vi "ZernikeModeAmp_RangeLimiter_v02.vi"(1 "x_in":dbl[](array[numeric]), 2 "Base Values":dbl[](array[numeric])) -> (0 "x_out":dbl[](array[numeric]))   [LabVIEW 2015]
panel:
  out "x_in relative":dbl[](array[numeric])
  in  "Limit":dbl[](array[numeric])=[1.0, 1.0, 1.0, 1.0, 1.5, 1.0, 1.5, 1.5, 1.0, 1.0, 1.0, 1.0, 1.0, 1.0, 1.0, 1.0, 1.0, 1.0, 1.0, 1.0, 1.0, 0.6, 1.0, 1.0, 1.0, 1.0, 1.0, 1.0, 1.0]
  # "piston"
  # "tip"
  # "tilt"
  # "defocus"
  # "astigmatism (oblique)"
  # "astigmatism (vertical)"
  # "coma"
  # "coma"
  # "trefoil (vertical)"
  # "trefoil (horizontal)"
  # "1st order Spherical Aberration"
  # "2nd order Astigmatism"
  # "2nd order Astigmatism"
  # "quadrafoil"
  # "quadrafoil"
  # "2nd order coma"
  # "2nd order coma"
  # "2nd order Spherical Aberration"
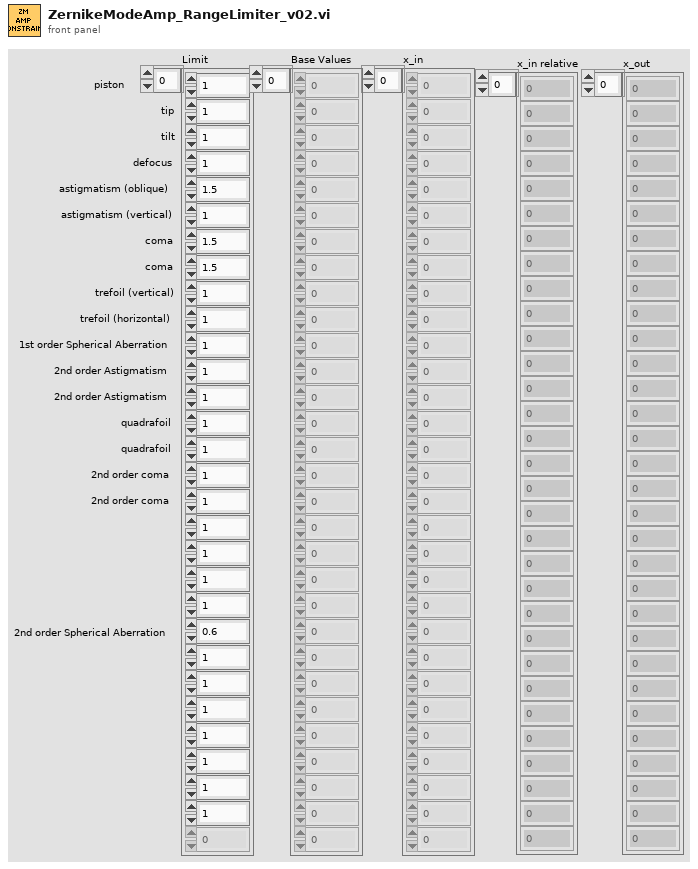
[diagram p1: front panel]
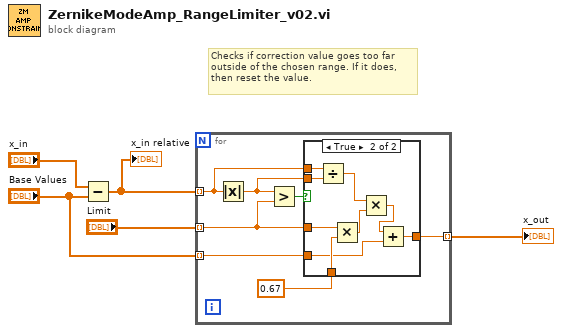
[diagram p0: block diagram]
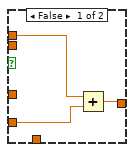
[diagram p2: hidden frame]
diagram:
  # "Checks if correction value goes too far \noutside of the chosen range. If it does, \nthen reset the value."
  n1 = Subtract(x="x_in", y="Base Values") -> (x-y=w3:dbl[])
  "x_in relative" <- w3
  n2 = for {
    tunnel: w3 -> [w11] mode=indexing
    tunnel: [w9] -> w5 mode=indexing
    tunnel: "Limit" -> [w7] mode=indexing
    tunnel: "Base Values" -> [w6] mode=indexing
    n3 = Absolute Value(x=w11) -> (abs(x)=w8:dbl)
    n4 = Greater?(x=w8, y=w7) -> (0:w12:bool)
    n5 = case shown="True" w12 {
      tunnel: w11 -> [w13 w22]
      tunnel: w8 -> [_ w21]
      tunnel: w7 -> [_ w20]
      tunnel: 0.67 ("y") -> [_ w19]
      tunnel: [w15 w16] -> w9
      tunnel: w6 -> [w14 w18]
      frame False {
        n6 = Add(x=w13, y=w14) -> (x+y=w15:dbl)
      }
      frame True {
        n7 = Divide(x=w22, y=w21) -> (x/y=w24:dbl)
        n8 = Multiply(x=w20, y=w19) -> (x*y=w23:dbl)
        n9 = Multiply(x=w24, y=w23) -> (x*y=w17:dbl)
        n10 = Add(x=w17, y=w18) -> (x+y=w16:dbl)
      }
    }
  }
  "x_out" <- w5
